vi "AccelerometerRequest.vi"(1 "FPGA I/O In":refnum<k21>="AccelerometerAB/AI0") -> ()   [LabVIEW 2016]
uses:
  <vilib>/rvi/eio/common/nirviEmuTemplateMethod_errors.vi
  <vilib>/rvi/interface/RandomDataEmulation/niFpgaRandomDataHandleErrors.vi
  <vilib>/eio/EIONode/EIONode.xnode
  <vilib>/rvi/DataTransferAndStorage/Container/XNode/niFpgaContainer.xnode
  <vilib>/rvi/interface/RandomDataEmulation/nirviRandomDataFpgaReadWriteTemplate.vi
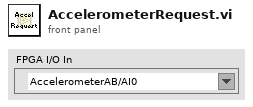
[diagram p1: front panel]
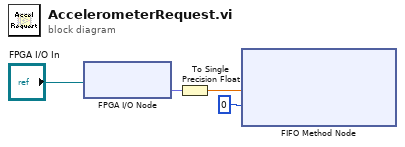
[diagram p0: block diagram]
diagram:
  n1 = xnode "FPGA I/O Node"("FPGA I/O In"="FPGA I/O In") -> ("I/O Item"=w4:fxp<+/-,24,5>)  [unwired: 1 out]
  n2 = To Single Precision Float(number=w4) -> (single precision float=w3:sgl)
  n3 = xnode ("FIFO Method Node")("Element"=w3, "Timeout"=0) -> ()  [unwired: 1 in, 2 out]
